vi "RUSHShooter.vi"(6 "Shooter Dial Delta":dbl, 7 "Shooter File Array":dbl[][](array[numeric]), 8 "Target Distance":dbl, 9 "Lock On Lights":dbl, 10 "Current Default Speed":dbl, 11 "Shooter Primed":bool) -> (3 "Shooter Output":dbl)   [LabVIEW 2011]
panel:
  in  "Dial Shooter Calibration Max Volt":dbl=3.3
  in  "Dial Shooter Calibration Min Volt":dbl
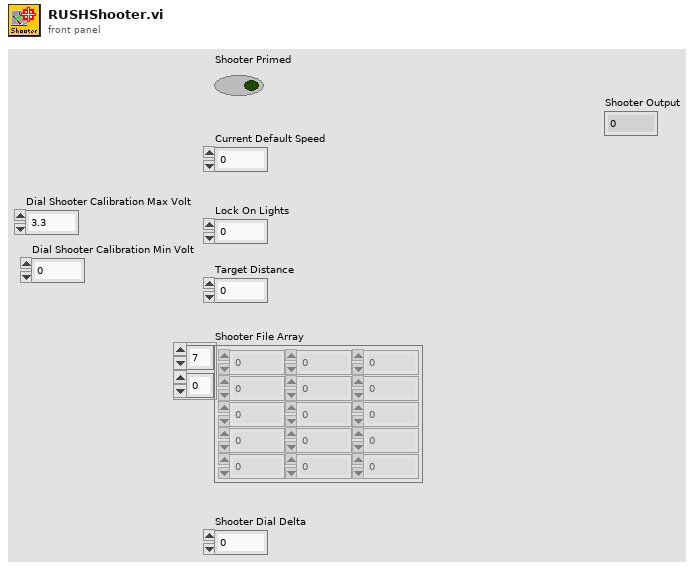
[diagram p1: front panel]
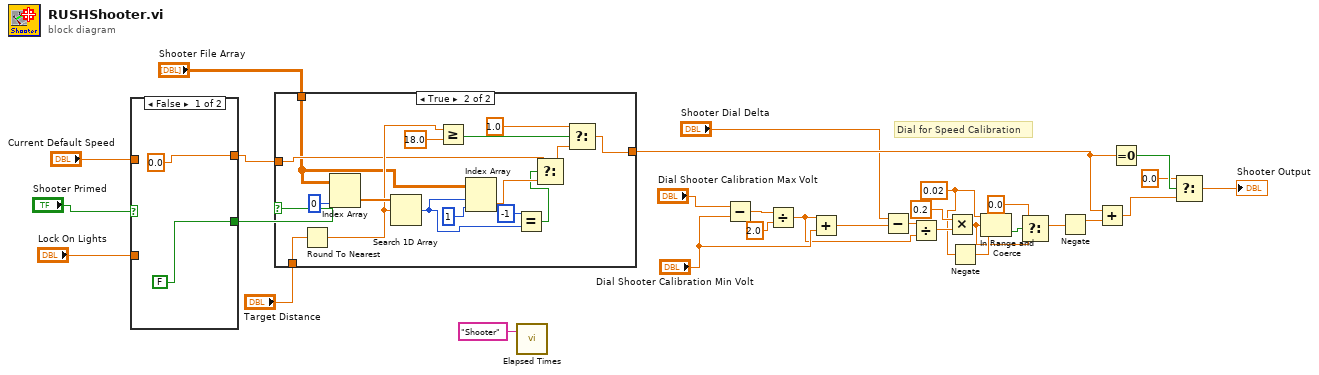
[diagram p0: block diagram]
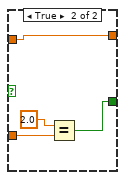
[diagram p3: hidden frame]
diagram:
  w17 = 0.02
  # "Dial for Speed Calibration"
  n1 = case shown="False" "Shooter Primed" {
    tunnel: [FALSE ("Shooter Primed") w35] -> w29
    tunnel: [0.0 w34] -> w30
    tunnel: "Current Default Speed" -> [_ w34]
    tunnel: "Lock On Lights" -> [_ w33]
    frame False {
    }
    frame True {
      n2 = Equal?(x=2.0, y=w33) -> (x = y?=w35:bool)
    }
  }
  n3 = case shown="True" w29 {
    tunnel: [w37 w48] -> w28
    tunnel: w30 -> [w37 w40]
    tunnel: "Shooter File Array" -> [_ w39]
    tunnel: "Target Distance" -> [_ w38]
    frame False {
    }
    frame True {
      n4 = Round To Nearest(number=w38) -> (nearest integer value=w49:dbl)
      n5 = Index Array(array=w39, index (col)=0 ("disabled index (col)")) -> (element=w51:dbl[])  [unwired: 1 in]
      n6 = Search 1D Array(1D array=w51, element=w49) -> (index of element=w43:i32)  [unwired: 1 in]
      n7 = Greater Or Equal?(x=w49, y=18.0) -> (x >= y?=w47:bool)
      n8 = Index Array(array=w39, index (row)=w43, index (col)=1 ("disabled index (col)")) -> (element=w44:dbl)
      n9 = Equal?(x=-1, y=w43) -> (x = y?=w41:bool)
      n10 = Select(t=w40, s=w41, f=w44) -> (s? t:f=w45:dbl)
      n11 = Select(t=1.0, s=w47, f=w45) -> (s? t:f=w48:dbl)
    }
  }
  n12 = call "Elapsed Times.vi"("Call Name"="Shooter") -> ()  [unwired: 2 in, 1 out]
  n13 = Subtract(x="Dial Shooter Calibration Max Volt", y="Dial Shooter Calibration Min Volt") -> (x-y=w26:dbl)
  n14 = Divide(x=w26, y=2.0) -> (x/y=w21:dbl)
  n15 = Add(x=w21, y="Dial Shooter Calibration Min Volt") -> (x+y=w23:dbl)
  n16 = Subtract(x="Shooter Dial Delta", y=w23) -> (x-y=w22:dbl)
  n17 = Divide(x=w22, y=w21) -> (x/y=w20:dbl)
  n18 = Multiply(x=0.2, y=w20) -> (x*y=w14:dbl)
  n19 = Negate(x=w17) -> (-x=w18:dbl)
  n20 = In Range and Coerce(upper limit=w17, x=w14, lower limit=w18) -> (In Range?=w16:bool)  [unwired: 1 out]
  n21 = Select(t=0.0, s=w16, f=w14) -> (s? t:f=w13:dbl)
  n22 = Negate(x=w13) -> (-x=w12:dbl)
  n23 = Add(x=w28, y=w12) -> (x+y=w10:dbl)
  n24 = Equal To 0?(x=w28) -> (x = 0?=w11:bool)
  n25 = Select(t=0.0, s=w11, f=w10) -> (s? t:f=→"Shooter Output":dbl)
